vi "Odbiór UDP z SbRIO.vi"(5 "Queue B in":T1, 8 "error in udp (no error)":errorcluster, 11 "port":refnum<k16>) -> (0 "error out udp":errorcluster, 1 "error out variant":errorcluster, 3 "UDP Network Connection out":refnum<k16>)   [LabVIEW 2015]
uses:
  QMH Fundamentals - Message Cluster.ctl
  CANFrameControl.ctl
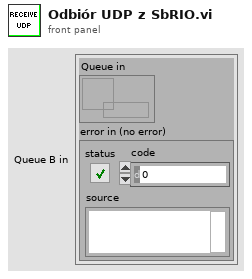
[diagram p1: front panel]
types:
  T1 = cluster{"Queue in":refnum<queue>, "error in (no error)":errorcluster}
  T2 = typedef "CANFrameControl.ctl" = cluster{"identifier":u32, "extended?":bool, "type":u8, "payload":u8[]}
  T3 = typedef "QMH Fundamentals - Message Cluster.ctl" = cluster{"Message":string, "Message Data":variant}
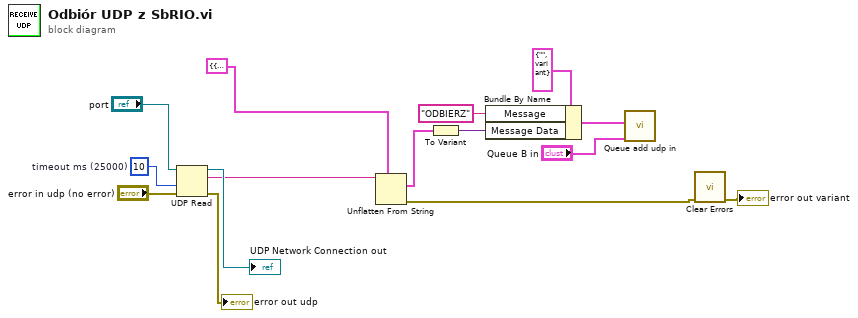
[diagram p0: block diagram]
diagram:
  w15 = 10  # timeout ms (25000)
  n1 = UDP Read(connection ID="port", timeout ms (25000)=w15, 8:"error in udp (no error)") -> (data out=w7:string, error out=→"error out udp":errorcluster, 3:→"UDP Network Connection out":refnum<k16>)  [unwired: 1 in, 2 out]
  n2 = Unflatten From String(type=cluster{"CAN frame":T2, "Delay":dbl} {"CAN frame"={"identifier"=0, "extended?"=FALSE, "type"=0, "payload"=[]}, "Delay"=0.0} ("output cluster"), binary string=w7) -> (value=w12:cluster{"CAN frame":T2, "Delay":dbl}, error out=w5:errorcluster)  [unwired: 3 in, 1 out]
  n3 = To Variant(anything=w12) -> (Variant=w11:variant)
  n4 = Bundle By Name(cluster=T3 {"Message"="", "Message Data"=variant} ("Message Cluster"), "Message"="ODBIERZ", "Message Data"=w11) -> (w2:T3)
  n5 = call "Queue add udp in.vi"("Queue B in"="Queue B in", "Message Cluster"=w2) -> ()  [unwired: 10 in]
  n6 = call <vilib>:"Clear Errors.vi"("error in (no error)"=w5) -> ("error out"=→"error out variant":errorcluster)  [unwired: 5 in, 1 out]
